vi "LVFPGA Rx.vi"(0 "device name":string="RIO0", 1 "Enabled Channels":string(combo)="0", 5 "IQ rate":dbl=10000000.0 caption="IQ Rate" format="%#.3pS/s", 7 "number of samples":i64=16834 caption="Number of Samples", 9 "run duration":dbl=5.0 format="%#_13g", 11 "error in":errorcluster) -> (6 "Coerced IQ Rate":dbl format="%#_6p", 8 "underflow":bool, 10 "overflow":bool, 15 "error out":errorcluster)   [LabVIEW 2014]
doc: "This template is for the Simple NI-USRP Streaming design, a design that shows the basics of streaming data from an NI USRP-294x/295x device. Refer to the block diagram for more information about how to use this template."
uses:
  subVIs/Start Trigger.ctl
  subVIs/Configure Signal (Level).vi
panel:
  out "Elements Remaining":u32 format="%0#8.0f"
  in  "host FIFO depth":u32=1000000
  out "pre-clear error":errorcluster
  in  "number of samples is finite":bool
  in  "stop":bool
  # "Rx Streaming"
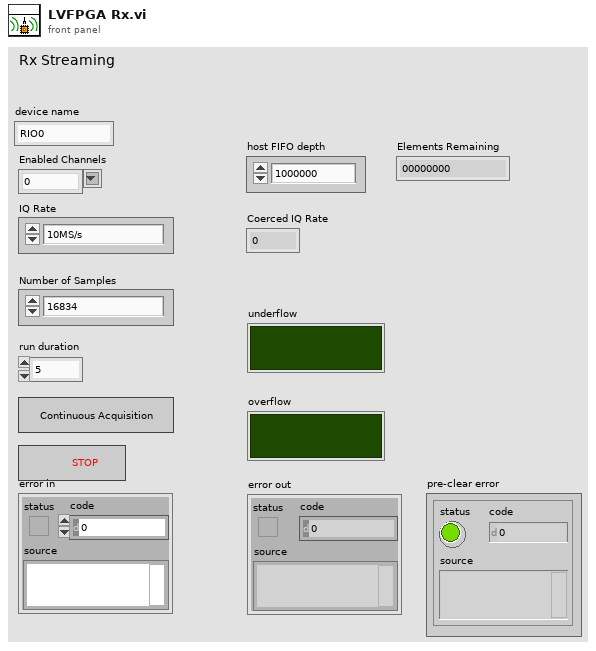
[diagram p1: front panel]
types:
  T1 = typedef "Start Trigger.ctl" = enum8{"Software", "Digital Edge", "Rx Start Trigger", "Tx Start Trigger", "Immediate"}
  T2 = cluster{"antenna":string, "frequency":dbl, "lo frequency":dbl, "level":dbl}[]
  T3 = typedef "niUsrpRio Config v1 Host.lvlib/niUsrpRio Session.ctl" = cluster{"Global Settings Register Bus":T4, "Radio 0 Settings Register Bus":T4, "Rx NI-USRP session":refnum<k15>, "Tx NI-USRP session":refnum<k15>, "FPGA Interface":refnum<k20>, "RIO Interface Number":u32, "EEPROM Header":T5, "Device Data Header":T6, "EEPROM Characterization Header":T7, "Characterization Data":T8[], "Characterization Data Valid?":bool, "Radio 1 Settings Register Bus":T4, "Radio Settings Bus Semaphore":T10, "FPGA Current Version":u32, "FPGA Oldest Compatible Version":u32, "Fixed Logic Current Version":u32, "Fixed Logic Oldest Compatible Version":u32, "FPGA Radio Settings Bus Current Version":u32, "FPGA Radio Settings Bus Oldest Compatible Version":u32}
  T4 = typedef "niInstr Register Bus v0 Host.lvlib/Register Bus Session.ctl" = refnum<queue>
  T5 = typedef "niUsrpRio Config v1 Host.lvlib/EEPROM Header.ctl" = cluster{"Checksum":u32, "Product Code":u16, "Hardware Current Version":u16, "Hardware Oldest Compatible Version":u16, "EEPROM Map Current Version":u16, "EEPROM Map Oldest Compatible Version":u16, "User Password":string, "Pointer to Factory Header":u32, "Pointer to User Header":u32, "Recommended Interval":u16, "Number of Reserved Bytes":i32, "Number of Daughterboards":u8, "Daughterboard IDs":u16[], "Daughterboard Serial Numbers":string[]}
  T6 = typedef "niUsrpRio Config v1 Host.lvlib/EEPROM Device Data Header.ctl" = cluster{"Checksum":u32, "Number of Channels":u8, "Number of Gain Settings":u16[], "Pointer to Characterization Data":u32[], "Number of Reserved Bytes":i32, "Number of Frequencies":u16[]}
  T7 = typedef "niUsrpRio Config v1 Host.lvlib/EEPROM Characterization Header.ctl" = cluster{"Checksum":u32, "Date":timestamp, "Temperature":sgl, "Misc. Info":string, "Pointer to Device Data Header":u32, "Number of Reserved Bytes":i32}
  T8 = typedef "niUsrpRio Config v1 Host.lvlib/Characterization Data.ctl" = cluster{"Gains[dB]":dbl[], "Frequencies [Hz]":dbl[], "IQ Imbalance Table":T9[], "Measured Gains[dB]":dbl[][]}
  T9 = typedef "niUsrpRio Config v1 Host.lvlib/IQ Imbalance.ctl" = cluster{"Gain Imbalance [linear]":dbl, "Phase Imbalance [radians]":dbl, "Offset":cdb}
  T10 = typedef "Semaphore RefNum" = refnum<k1>
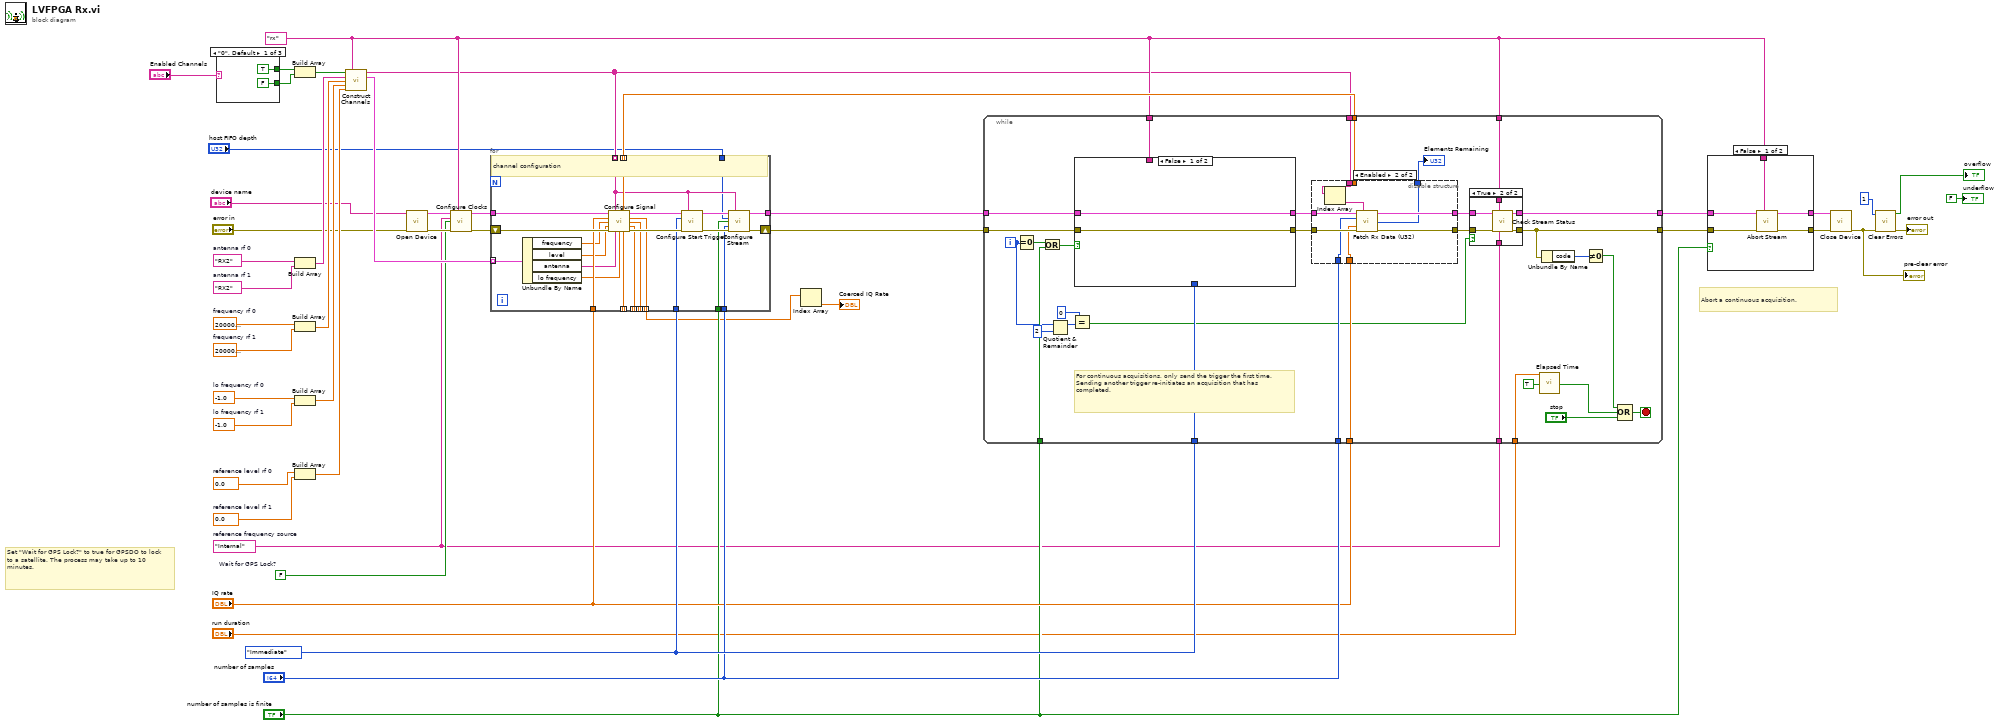
[diagram p0: block diagram]
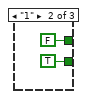
[diagram p2: hidden frame]
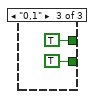
[diagram p3: hidden frame]
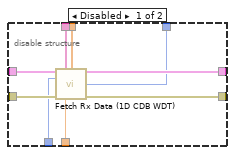
[diagram p6: hidden frame]
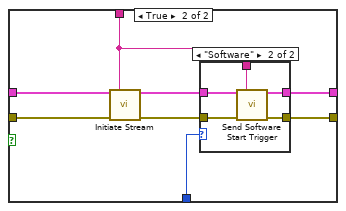
[diagram p7: hidden frame]
diagram:
  w46 = Start_Trigger."Immediate" ("start trigger")
  w14 = "Internal"  # reference frequency source
  w31 = 0.0  # reference level rf 1
  w30 = 0.0  # reference level rf 0
  w32 = -1.0  # lo frequency rf 1
  w33 = -1.0  # lo frequency rf 0
  w34 = 2000000000.0  # frequency rf 1
  w35 = 2000000000.0  # frequency rf 0
  w38 = "RX2"  # antenna rf 1
  w37 = "RX2"  # antenna rf 0
  w15 = FALSE  # Wait for GPS Lock?
  w23 = "rx" ("scope")
  # "Set \"Wait for GPS Lock?\" to true for GPSDO to lock to a satellite. The process may take up to 10 minutes."
  # "Abort a continuous acquisition."
  n1 = case shown="\"0\", Default" "Enabled Channels" {
    tunnel: [TRUE FALSE TRUE] -> w12
    tunnel: [FALSE TRUE TRUE] -> w11
    frame "0", Default {
    }
    frame "1" {
    }
    frame "0,1" {
    }
  }
  n2 = Build Array(w12, w11) -> (w36:bool[])
  n3 = Build Array(w37, w38) -> (w28:string[])
  n4 = Build Array(w35, w34) -> (w27:dbl[])
  n5 = Build Array(w33, w32) -> (w26:dbl[])
  n6 = Build Array(w30, w31) -> (w25:dbl[])
  n7 = call "Construct Channels.vi"("enabled channels"=w36, "scope"=w23, "antennas"=w28, "frequencies"=w27, "lo frequencies"=w26, "levels"=w25) -> ("channels"=w22:string[], "channel configurations"=w24:T2)  [unwired: 8 in]
  n8 = call "Open Device.vi"("USRP RIO device"="device name", "error in"="error in") -> ("niUsrpRio Session (out)"=w21:T3, "error out"=w20:errorcluster)  [unwired: 12 in]
  n9 = call "Configure Clocks.vi"("niUsrpRio Session"=w21, "scope"=w23, "Reference Frequency Source"=w14, "Wait for GPS Lock?"=w15, "error in"=w20) -> ("niUsrpRio Session (out)"=w19:T3, "error out"=w18:errorcluster)  [unwired: 9 in]
  n10 = for {
    tunnel: [w64] -> _ mode=indexing
    tunnel: [w75] -> w17
    tunnel: w46 -> [w74]
    tunnel: w19 -> [w69]
    tunnel: [w68] -> w45 mode=indexing
    tunnel: "number of samples" -> [w67]
    tunnel: "number of samples is finite" -> [w66]
    shift-right: [w76] -> w47
    shift-left: w18 -> [w70]
    tunnel: "IQ rate" -> [w65]
    tunnel: [w63] -> _ mode=indexing
    tunnel: [w62] -> _ mode=indexing
    tunnel: [w61] -> w9 mode=indexing
    tunnel: w24 -> [w60] mode=indexing
    tunnel: w22 -> [w55] mode=indexing
    tunnel: "host FIFO depth" -> [w54]
    # "channel configuration"
    n11 = Unbundle By Name(w60) -> ("frequency"=w59:dbl, "level"=w56:dbl, "antenna"=w58:string, "lo frequency"=w57:dbl)
    n12 = call-poly "Configure Signal.vi"("niUsrpRio Session"=w69, "scope"=w55, "sample rate [S/s]"=w65, "frequency [Hz]"=w59, "level [dBm]"=w56, "error in"=w70, "Active Antenna"=w58, "LO frequency [Hz]"=w57) -> ("coerced vertical range [Vpp]"=w68:dbl, "niUsrpRio Session (out)"=w72:T3, "coerced sample rate [S/s]"=w61:dbl, "coerced frequency [Hz]"=w62:dbl, "coerced level [dBm]"=w63:dbl, "coerced LO frequency [Hz]"=w64:dbl, "error out"=w77:errorcluster)  [unwired: 1 in]
    n13 = call "Configure Start Trigger.vi"("niUsrpRio Session"=w72, "scope"=w55, "start trigger"=w74, "error in"=w77) -> ("niUsrpRio Session (out)"=w71:T3, "error out"=w73:errorcluster)  [unwired: 10 in]
    n14 = call "Configure Stream.vi"("niUsrpRio Session"=w71, "scope"=w55, "host FIFO depth"=w54, "number of samples is finite"=w66, "number of samples"=w67, "error in"=w73) -> ("niUsrpRio Session (out)"=w75:T3, "error out"=w76:errorcluster)  [unwired: 8 in]
  }
  n15 = Index Array(array=w9) -> (element=→"Coerced IQ Rate":dbl)  [unwired: 1 in]
  n16 = while {
    tunnel: w17 -> [w104]
    tunnel: [w108] -> w43
    tunnel: w45 -> [w98]
    tunnel: "IQ rate" -> [w102]
    tunnel: "number of samples" -> [w101]
    tunnel: w46 -> [w107]
    tunnel: w47 -> [w106]
    tunnel: [w86] -> w42
    tunnel: "number of samples is finite" -> [w99]
    tunnel: w23 -> [w96]
    tunnel: w23 -> [w95]
    tunnel: w22 -> [w94]
    tunnel: w14 -> [w91]
    tunnel: "run duration" -> [w87]
    i -> [w82]
    stop <- w109 stop-if-true
    # "For continuous acquisitions, only send the trigger the first time. Sending another trigger re-initiates an acquisition that has completed."
    # "Acquire and Fetch a waveform"
    n17 = Equal To 0?(x=w82) -> (x = 0?=w100:bool)
    n18 = Or(x=w100, y=w99) -> (x .or. y?=w97:bool)
    n19 = Quotient & Remainder(x=w82, y=2) -> (x-y*floor(x/y)=w80:i32)  [unwired: 1 out]
    n20 = Equal?(x=0, y=w80) -> (x = y?=w79:bool)
    n21 = case shown="False" w97 {
      tunnel: w107 -> [_ w141]
      tunnel: w106 -> [w137 w145]
      tunnel: [w137 w143] -> w105
      tunnel: w104 -> [w136 w139]
      tunnel: [w136 w138] -> w103
      tunnel: w95 -> [_ w140]
      frame False {
      }
      frame True {
        n22 = call "Initiate Stream.vi"("niUsrpRio Session"=w139, "scope"=w140, "error in"=w145) -> ("niUsrpRio Session (out)"=w142:T3, "error out"=w144:errorcluster)  [unwired: 11 in]
        n23 = case shown="\"Software\"" w141 {
          tunnel: w144 -> [w147 w152]
          tunnel: [w147 w151] -> w143
          tunnel: w142 -> [w146 w150]
          tunnel: w140 -> [_ w149]
          tunnel: [w146 w148] -> w138
          frame Default {
          }
          frame "Software" {
            n24 = call "Send Software Start Trigger.vi"("niUsrpRio Session"=w150, "scope"=w149, "error in"=w152) -> ("niUsrpRio Session (out)"=w148:T3, "error out"=w151:errorcluster)  [unwired: 11 in]
          }
        }
      }
    }
    n25 = disable-structure shown="Enabled" {
      disable-tunnel: w105 -> [w126 w134]
      disable-tunnel: w103 -> [w125 w135]
      disable-tunnel: w102 -> [w124 w128]
      disable-tunnel: w101 -> [w123 w129]
      disable-tunnel: w98 -> [w122 _]
      disable-tunnel: w94 -> [w121 w131]
      disable-tunnel: [w120 w132] -> w93
      disable-tunnel: [w119 w133] -> w92
      disable-tunnel: [w118 w127] -> w83
      frame Disabled {
        n26 = call "Fetch Rx Data (1D CDB WDT).vi"("niUsrpRio Session"=w125, "scope"=w121, "vertical ranges [Vpp]"=w122, "number of samples"=w123, "error in"=w126, "sample rate"=w124) -> ("niUsrpRio Session (out)"=w119:T3, "elements remaining"=w118:u32, "error out"=w120:errorcluster)  [unwired: 6 in, 1 out]
      }
      frame Enabled {
        n27 = Index Array(array=w131) -> (element=w130:string)  [unwired: 1 in]
        n28 = call "Fetch Rx Data (U32).vi"("niUsrpRio Session"=w135, "scope"=w130, "number of samples"=w129, "timeout"=w128, "error in"=w134) -> ("niUsrpRio Session (out)"=w133:T3, "Elements Remaining"=w127:u32, "error out"=w132:errorcluster)  [unwired: 6 in, 2 out]
      }
    }
    "Elements Remaining" <- w83
    n29 = case shown="True" w79 {
      tunnel: [w110 w117] -> w108
      tunnel: w96 -> [_ w116]
      tunnel: w93 -> [w111 w115]
      tunnel: w92 -> [w110 w114]
      tunnel: w91 -> [_ w113]
      tunnel: [w111 w112] -> w86
      frame False {
      }
      frame True {
        n30 = call "Check Stream Status.vi"("niUsrpRio Session"=w114, "scope"=w116, "error in"=w115, "reference frequency source"=w113) -> ("niUsrpRio Session (out)"=w117:T3, "error out"=w112:errorcluster)  [unwired: 9 in, 1 out]
      }
    }
    n31 = call "Elapsed Time"("Time Target (s)"=w87, "Auto Reset"=TRUE) -> ("Time has Elapsed"=w89:bool)  [unwired: 10 in, 7 out]
    n32 = Unbundle By Name(w86) -> ("code"=w85:i32)
    n33 = Not Equal To 0?(x=w85) -> (x != 0?=w84:bool)
    n34 = Compound Arithmetic op=OR(w84, w89, "stop") -> (w109:bool)
  }
  n35 = case shown="False" "number of samples is finite" {
    tunnel: w43 -> [w157 w159]
    tunnel: w42 -> [w156 w158]
    tunnel: [w155 w159] -> w41
    tunnel: [w154 w158] -> w40
    tunnel: w23 -> [w153 _]
    frame False {
      n36 = call "Abort Stream.vi"("niUsrpRio Session"=w157, "scope"=w153, "error in"=w156) -> ("niUsrpRio Session (out)"=w155:T3, "error out"=w154:errorcluster)  [unwired: 11 in]
    }
    frame True {
    }
  }
  n37 = call "Close Device.vi"("niUsrpRio Session"=w41, "error in"=w40) -> ("error out"=w7:errorcluster)  [unwired: 13 in]
  "pre-clear error" <- w7
  n38 = call <vilib>:"Clear Errors.vi"("error in (no error)"=w7, "specific error code to clear (0: all)"=1) -> ("error out"=→"error out":errorcluster, "specific error cleared?"=→"overflow":bool)  [unwired: 4 in]
  "underflow" <- FALSE ("underflow")
